vi "SQL_EDITOR_prepare_UPDATE_statement.vi"(7 "nmb_of_top_rows (all)":i32, 8 "error_in":errorcluster, 10 "selected_record":i32, 11 "REF_EDIT_records":string[][](array[string])) -> (0 "error_out":errorcluster, 3 "UPDATE_statement":string)   [LabVIEW 2019]
uses:
  FGV/SQL_EDITOR_records_display/FGV_SQL_EDITOR_records_display.ctl
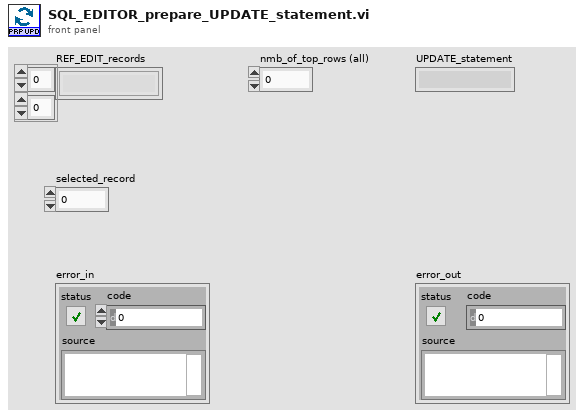
[diagram p1: front panel]
types:
  T1 = typedef "FGV_SQL_EDITOR_records_display.ctl" = enum16{"initialize", "set_table_name", "set_column_name", "set_value_to_select", "set_order_by", "set_asc_desc", "set_headers", "set_records", "get_table_name", "get_column_name", "get_value_to_select", "get_headers", "get_all_info", "record_added?", "record_inserted?", "record_edited?", "record_updated?", "record_deleted?", "discard_changes"}
  T2 = typedef "SQL_EDITOR_all_info.ctl" = cluster{"table":string, "column":string, "value_to_select":string, "order_by":string, "asc_desc":string, "headers":string[], "uneditable_columns":string[], "uneditable_columns":i32[], "editable_columns":i32[], "values_in_database":string[][], "size":cluster{"columns":i32, "SQL_rows":i32, "disp_rows":i32}, "SQL_record_states":T3[]}
  T3 = typedef "SQL_record_states.ctl" = enum16{"Equal", "Added", "Edited", "Deleted"}
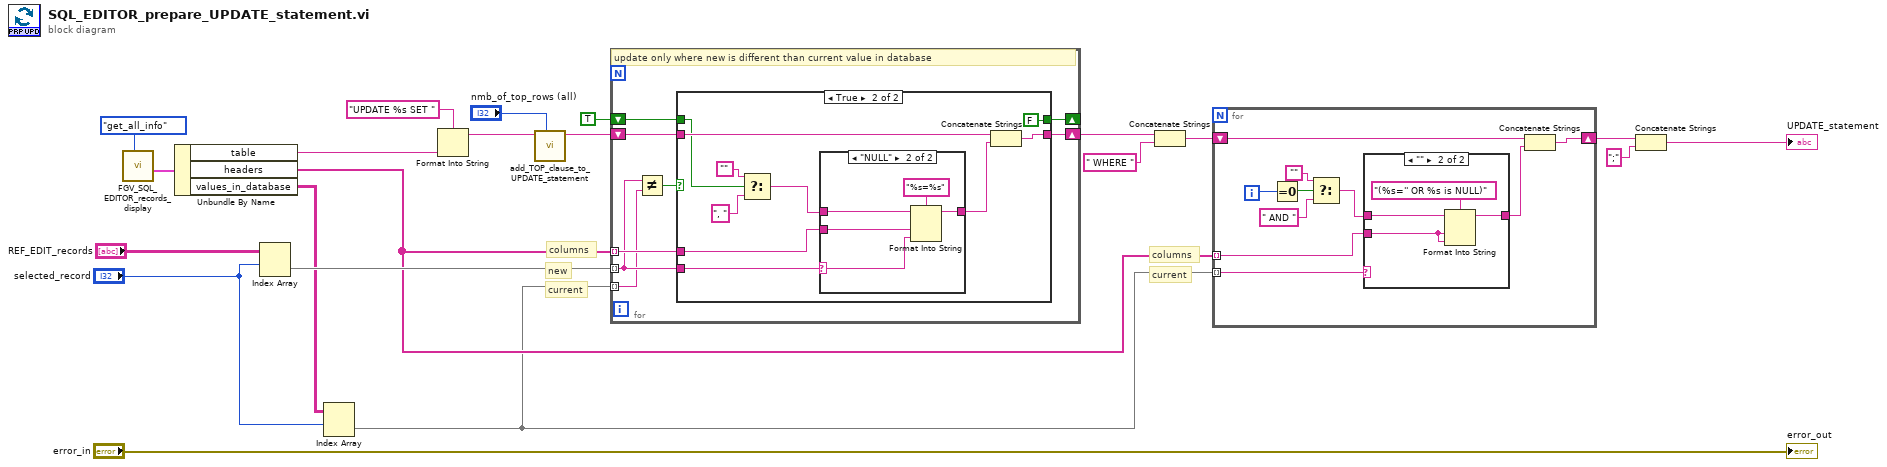
[diagram p0: block diagram]
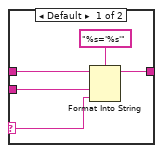
[diagram p2: hidden frame]
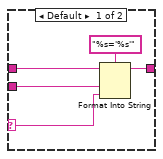
[diagram p4: hidden frame]
diagram:
  # "current"
  # "current"
  # "columns"
  # "new"
  # "columns"
  n1 = call "FGV_SQL_EDITOR_records_display.vi"("options"=FGV_SQL_EDITOR_records_display."get_all_info") -> ("all_info"=w9:T2)  [unwired: 7 in, 3 out]
  n2 = Unbundle By Name(w9) -> ("table"=w8:string, "headers"=w4:string[], "values_in_database"=w3:string[][])
  n3 = Index Array(array="REF_EDIT_records", index (row)="selected_record") -> (element=w5:string[])  [unwired: 1 in]
  n4 = Index Array(array=w3, index (row)="selected_record") -> (element=w2:string[])  [unwired: 1 in]
  n5 = Format Into String(format string="UPDATE %s SET ", w8) -> (resulting string=w13:string)  [unwired: 2 in, 1 out]
  n6 = call "add_TOP_clause_to_UPDATE_statement.vi"("nmb_of_top_rows (all)"="nmb_of_top_rows (all)", "UPDATE_statement_in"=w13) -> ("UPDATE_statement_out"=w12:string)  [unwired: 8 in, 1 out]
  n7 = for {
    shift-right: [w28] -> w21
    shift-left: w12 -> [w29]
    tunnel: w4 -> [w27] mode=indexing
    tunnel: w5 -> [w25] mode=indexing
    tunnel: w2 -> [w24] mode=indexing
    shift-right: [w22] -> _
    shift-left: TRUE -> [w23]
    # "update only where new is different than current value in database"
    n8 = Not Equal?(x=w25, y=w24) -> (x != y?=w26:bool)
    n9 = case shown="True" w26 {
      tunnel: w29 -> [w31 w39]
      tunnel: [w31 w36] -> w28
      tunnel: w27 -> [_ w35]
      tunnel: w25 -> [_ w34]
      tunnel: w23 -> [w30 w33]
      tunnel: [w30 FALSE] -> w22
      frame False {
      }
      frame True {
        n10 = Select(t="", s=w33, f=", ") -> (s? t:f=w38:string)
        n11 = case shown="\"NULL\"" w34 {
          selector: w34 -> [w42 w47]
          tunnel: w38 -> [w45 w50]
          tunnel: [w44 w49] -> w37
          tunnel: w35 -> [w43 w48]
          frame Default {
            n12 = Format Into String(format string="%s='%s'", initial string=w45, w43, w42) -> (resulting string=w44:string)  [unwired: 1 in, 1 out]
          }
          frame "NULL" {
            n13 = Format Into String(format string="%s=%s", initial string=w50, w48, w47) -> (resulting string=w49:string)  [unwired: 1 in, 1 out]
          }
        }
        n14 = Concatenate Strings(w39, w37) -> (w36:string)
      }
    }
  }
  n15 = Concatenate Strings(w21, " WHERE ") -> (w19:string)
  n16 = for {
    shift-right: [w54] -> w18
    shift-left: w19 -> [w57]
    tunnel: w4 -> [w53] mode=indexing
    tunnel: w2 -> [w52] mode=indexing
    i -> [w61]
    n17 = Equal To 0?(x=w61) -> (x = 0?=w60:bool)
    n18 = Select(t="", s=w60, f=" AND ") -> (s? t:f=w56:string)
    n19 = case shown="\"\"" w52 {
      selector: w52 -> [w62 _]
      tunnel: w56 -> [w65 w69]
      tunnel: [w64 w68] -> w55
      tunnel: w53 -> [w63 w67]
      frame Default {
        n20 = Format Into String(format string="%s='%s'", initial string=w65, w63, w62) -> (resulting string=w64:string)  [unwired: 1 in, 1 out]
      }
      frame "" {
        n21 = Format Into String(format string="(%s='' OR %s is NULL)", initial string=w69, w67, w67) -> (resulting string=w68:string)  [unwired: 1 in, 1 out]
      }
    }
    n22 = Concatenate Strings(w57, w55) -> (w54:string)
  }
  n23 = Concatenate Strings(w18, ";") -> (→"UPDATE_statement":string)
  "error_out" <- "error_in"
